vi "A_csapat_hang.vi"(10 "Index":i32, 11 "A csapat(1D tömb)":string[](array[string])) -> (1 "Becenév":string, 2 "\"A\" csapat játékosa":waveform(dbl)[](array[waveform]))   [LabVIEW 2013]
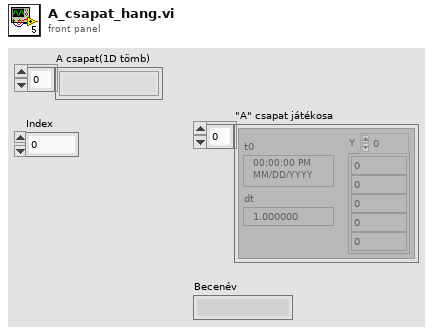
[diagram p1: front panel]
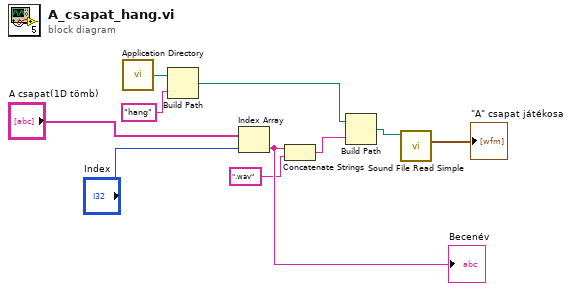
[diagram p0: block diagram]
diagram:
  n1 = call <vilib>:"Application Directory.vi"() -> ("Application Directory"=w3:path)
  n2 = Build Path(base path=w3, name or relative path="hang") -> (appended path=w10:path)
  n3 = Index Array(array="A csapat(1D tömb)", index="Index") -> (element=w8:string)
  "Becenév" <- w8
  n4 = Concatenate Strings(w8, ".wav" ("name or relative path")) -> (w5:string)
  n5 = Build Path(base path=w10, name or relative path=w5) -> (appended path=w7:path)
  n6 = call <vilib>:"Sound File Read Simple.vi"("path"=w7) -> ("data"=→"\"A\" csapat játékosa":waveform(dbl)[])  [unwired: 7 in, 3 out]
